vi "Exit if EXE.vi"(3 "error in (no error)":errorcluster, 5 "quit? (T)":bool=TRUE) -> (0 "error out":errorcluster)   [LabVIEW 2017]
doc: "Exit if current path includes EXE."
panel:
  # "Exit if current path includes EXE."
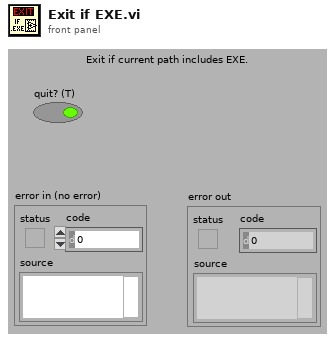
[diagram p1: front panel]
types:
  T1 = enum32{"invalid app kind", "Development System", "Run Time System", "Student Edition", "Embedded LabVIEW", "Evaluation", "Custom"}
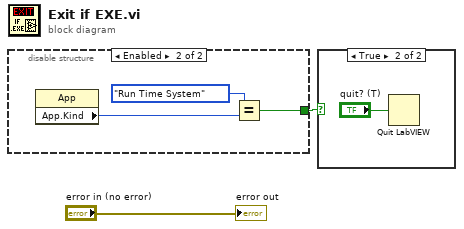
[diagram p0: block diagram]
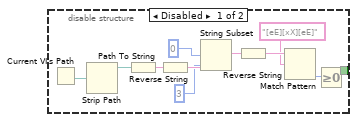
[diagram p2: hidden frame]
diagram:
  n1 = disable-structure shown="Enabled" {
    disable-tunnel: [w3 w14] -> w1
    frame Disabled {
      n2 = Current VI's Path() -> (path=w5:path)
      n3 = Strip Path(path=w5) -> (stripped path=w4:path)  [unwired: 1 out]
      n4 = Path To String(path=w4) -> (string=w13:string)
      n5 = Reverse String(1:w13) -> (0:w12:string)
      n6 = String Subset(string=w12, offset (0)=0, length (rest)=3 ("length")) -> (substring=w9:string)
      n7 = Reverse String(1:w9) -> (0:w8:string)
      n8 = Match Pattern(string=w8, regular expression="[eE][xX][eE]") -> (offset past match=w6:i32)  [unwired: 1 in, 3 out]
      n9 = Greater Or Equal To 0?(x=w6) -> (x >= 0?=w3:bool)
    }
    frame Enabled {
      n10 = property class="App"() -> ("App.Kind"=w16:T1)  [unwired: 2 in, 2 out]
      n11 = Equal?(x=T1."Run Time System" ("Application:Kind"), y=w16) -> (x = y?=w14:bool)
    }
  }
  n12 = case shown="True" w1 {
    frame False {
    }
    frame True {
      n13 = Quit LabVIEW(quit? (T)="quit? (T)") -> ()
    }
  }
  "error out" <- "error in (no error)"
